vi "LaunchSettingsPanel.vi"(7 "SettingQueue":refnum<queue>, 8 "error in (no error)":errorcluster, 9 "MainUI":refnum<queue>, 10 "Settings in":T1, 11 "Subpanel":refnum<vi>) -> (0 "error out":errorcluster)   [LabVIEW 2019, in "MainController.lvlib"]
uses:
  MainController.lvlib
  Settings/Cluster - Settings.ctl
  Cluster - HardwareConfiguration.ctl
  Cluster - TestSettings.ctl
  Cluster - MainControllerMessage.ctl
  Enum - MainState.ctl
  Settings/CTL_MessageCluster.ctl
  Settings/CTL_SettingsMessage.ctl
  Settings/Settings Panel.vi
  support/User Interface/UserInterface.lvlib
  Settings/Settings.lvlib
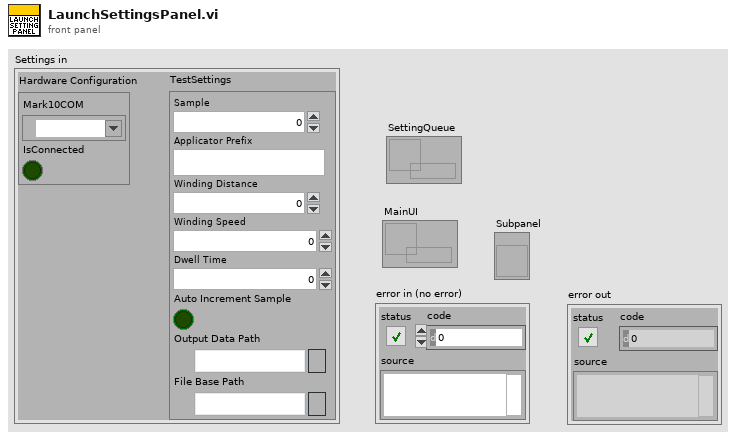
[diagram p1: front panel]
types:
  T1 = typedef "Settings.lvlib/Cluster - Settings.ctl" = cluster{"Hardware Configuration":T2, "TestSettings":T3}
  T2 = typedef "MainController.lvlib/Cluster - HardwareConfiguration.ctl" = cluster{"Mark10COM":refnum<visa-resource-name>, "IsConnected":bool}
  T3 = typedef "MainController.lvlib/Cluster - TestSettings.ctl" = cluster{"Sample":u32, "Applicator Prefix":string, "Winding Distance":dbl, "Winding Speed":dbl, "Dwell Time":dbl, "Auto Increment Sample":bool, "Output Data Path":path, "File Base Path":path}
  T4 = typedef "Settings.lvlib/CTL_SettingsMessage.ctl" = enum16{"Inititalize", "Idle", "LoadSettings", "SaveSettings", "Exit"}
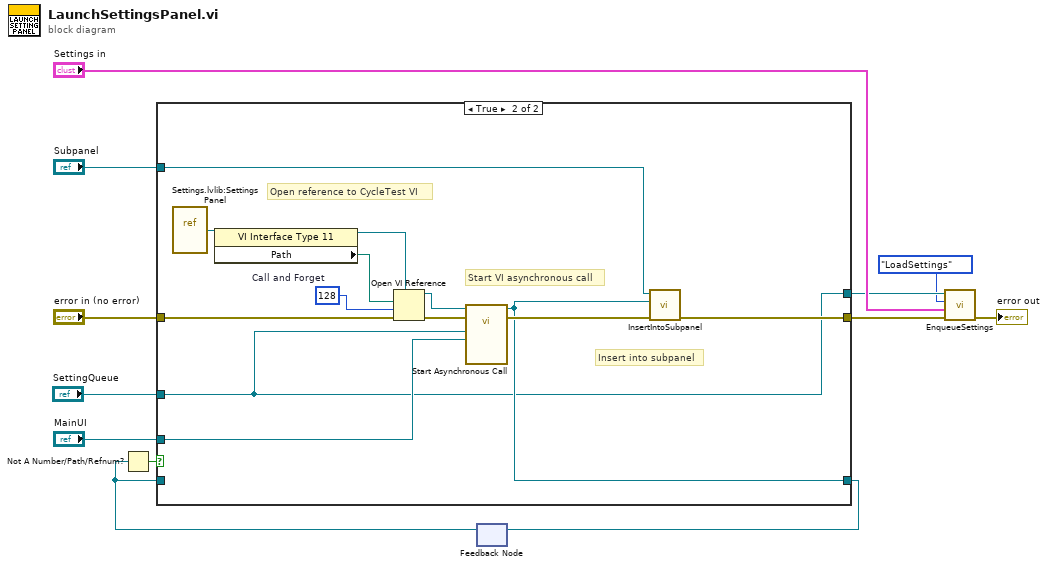
[diagram p0: block diagram]
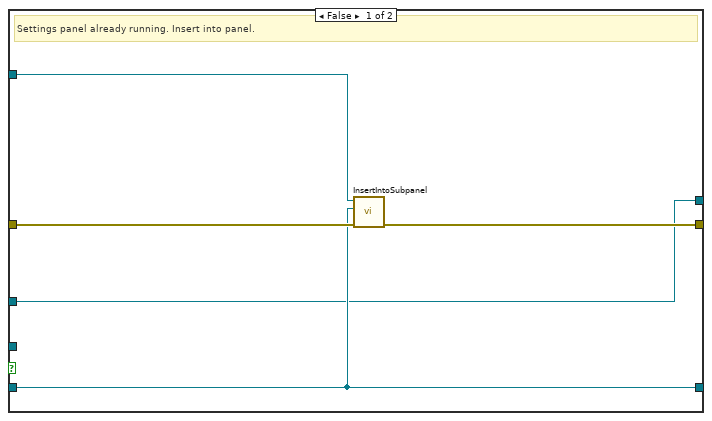
[diagram p2: hidden frame]
diagram:
  n1 = feedback #1() -> (w9:refnum<vi>)  [unwired: 1 in]
  n2 = Not A Number/Path/Refnum?(number/path/refnum=w9) -> (NaN/Path/Refnum?=w8:bool)
  n3 = case shown="True" w8 {
    tunnel: "error in (no error)" -> [w17 w30]
    tunnel: "Subpanel" -> [w16 w28]
    tunnel: [w14 w19] -> w5
    tunnel: [w15 w22] -> w10
    tunnel: w9 -> [w15 _]
    tunnel: "MainUI" -> [_ w20]
    tunnel: "SettingQueue" -> [w13 w18]
    tunnel: [w13 w18] -> w2
    frame False {
      # "Settings panel already running. Insert into panel."
      n4 = call "InsertIntoSubpanel.vi"("error in (no error)"=w17, "VI Ref"=w15, "Subpanel"=w16) -> ("error out"=w14:errorcluster)  [unwired: 8 in]
    }
    frame True {
      w24 = 128  # Call and Forget
      # "Insert into subpanel"
      # "Start VI asynchronous call"
      # "Open reference to CycleTest VI"
      n5 = vi-ref "Settings.lvlib:Settings Panel.vi"() -> (w25:refnum<vi>)
      n6 = property class="VI Interface Type 11"(reference=w25) -> (reference out=w21:refnum<vi>, "Path"=w29:path)  [unwired: 1 in, 1 out]
      n7 = Open VI Reference(type specifier VI Refnum (for type only)=w21, vi path=w29, options=w24, error in (no error)=w30) -> (vi reference=w27:refnum<vi>, error out=w26:errorcluster)  [unwired: 2 in]
      n8 = call-by-ref "Start Asynchronous Call"(reference=w27, error in=w26, "MainUI"=w20, "SettingQueue"=w18) -> (reference out=w22:refnum<vi>, error out=w23:errorcluster)  [unwired: 9 in, 1 out]
      n9 = call "InsertIntoSubpanel.vi"("error in (no error)"=w23, "VI Ref"=w22, "Subpanel"=w28) -> ("error out"=w19:errorcluster)  [unwired: 8 in]
    }
  }
  n10 = feedback-in #1(w10) -> ()
  n11 = call "EnqueueSettings.vi"("error in (no error)"=w5, "Data"="Settings in", "Message"=CTL_SettingsMessage."LoadSettings", "SettingsQueue"=w2) -> ("error out"=→"error out":errorcluster)  [unwired: 6 in, 1 out]
